vi "KH_DAQ_TURCK_StatusAO Write.vi"(11 "TBEN-S2-4AO Input Values":T1) -> (3 "Stauts AO":bool[](array[boolean]))   [LabVIEW 2021]
uses:
  KH Turck EthernetIP 17.12/KH TURCK ETHERNETIP TDefCluster TBEN-S2-4AO Input Values.ctl
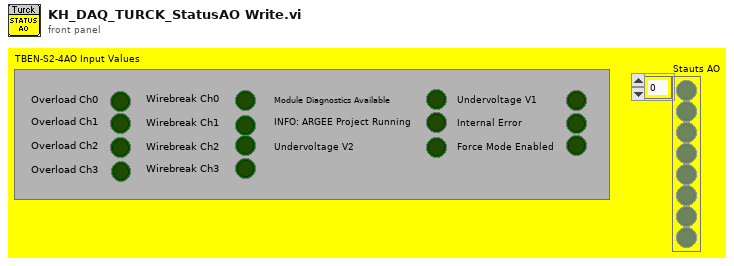
[diagram p1: front panel]
types:
  T1 = typedef "KH TURCK ETHERNETIP TDefCluster TBEN-S2-4AO Input Values.ctl" = cluster{"Overload Ch0":bool, "Overload Ch1":bool, "Overload Ch2":bool, "Overload Ch3":bool, "Wirebreak Ch0":bool, "Wirebreak Ch1":bool, "Wirebreak Ch2":bool, "Wirebreak Ch3":bool, "Module Diagnostics Available":bool, "INFO: ARGEE Project Running":bool, "Undervoltage V2":bool, "Undervoltage V1":bool, "Internal Error":bool, "Force Mode Enabled":bool}
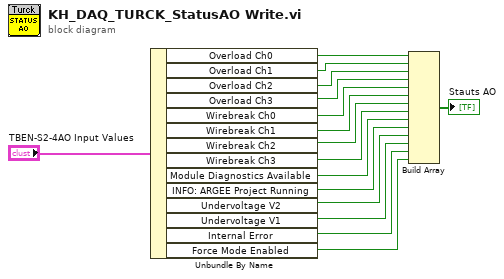
[diagram p0: block diagram]
diagram:
  n1 = Unbundle By Name("TBEN-S2-4AO Input Values") -> ("Overload Ch0"=w15:bool, "Overload Ch1"=w14:bool, "Overload Ch2"=w13:bool, "Overload Ch3"=w12:bool, "Wirebreak Ch0"=w11:bool, "Wirebreak Ch1"=w10:bool, "Wirebreak Ch2"=w9:bool, "Wirebreak Ch3"=w8:bool, "Module Diagnostics Available"=w7:bool, "INFO: ARGEE Project Running"=w6:bool, "Undervoltage V2"=w5:bool, "Undervoltage V1"=w4:bool, "Internal Error"=w3:bool, "Force Mode Enabled"=w2:bool)
  n2 = Build Array(w15, w14, w13, w12, w11, w10, w9, w8, w7, w6, w5, w4, w3, w2) -> (→"Stauts AO":bool[])
